vi "GUI_HTT_Cam_SubVI.vi"() -> (3 "image::2":T3(plugin-control))   [LabVIEW 2013]
uses:
  Shared/GUI_Template/GUI_master/tcp_new_data_event.ctl
  Shared/GUI_Template/GUI_master/tcp new data cluster.ctl
panel:
  in  "UDP error message":string
  out "tcp data event 2":T1
  out "error IO 2":errorcluster
  in  "active cams":string
  out "CCDs":string[](array[string])
  out "Cameras":T2
  in  "triggerdelay::2":dbl=0.001 caption="triggerdelay" min=0.0 max=10000.0 format="%_4p"
  in  "trigger::2":bool caption="Trigger"
  in  "exposure::2":dbl=0.001 caption="exposure" min=0.0001 max=1.0 format="%_4p"
  in  "GUIdevice 2":string="BellaCam13_4_gmode_s"
  out "tcp data event":T1
  in  "Refresh Button":bool caption="Update Crosshairs"
  in  "Select device":string(combo)="FrogHPD"
  in  "stop":bool
  in  "GUIdevice 1":string="HPD_CCD"
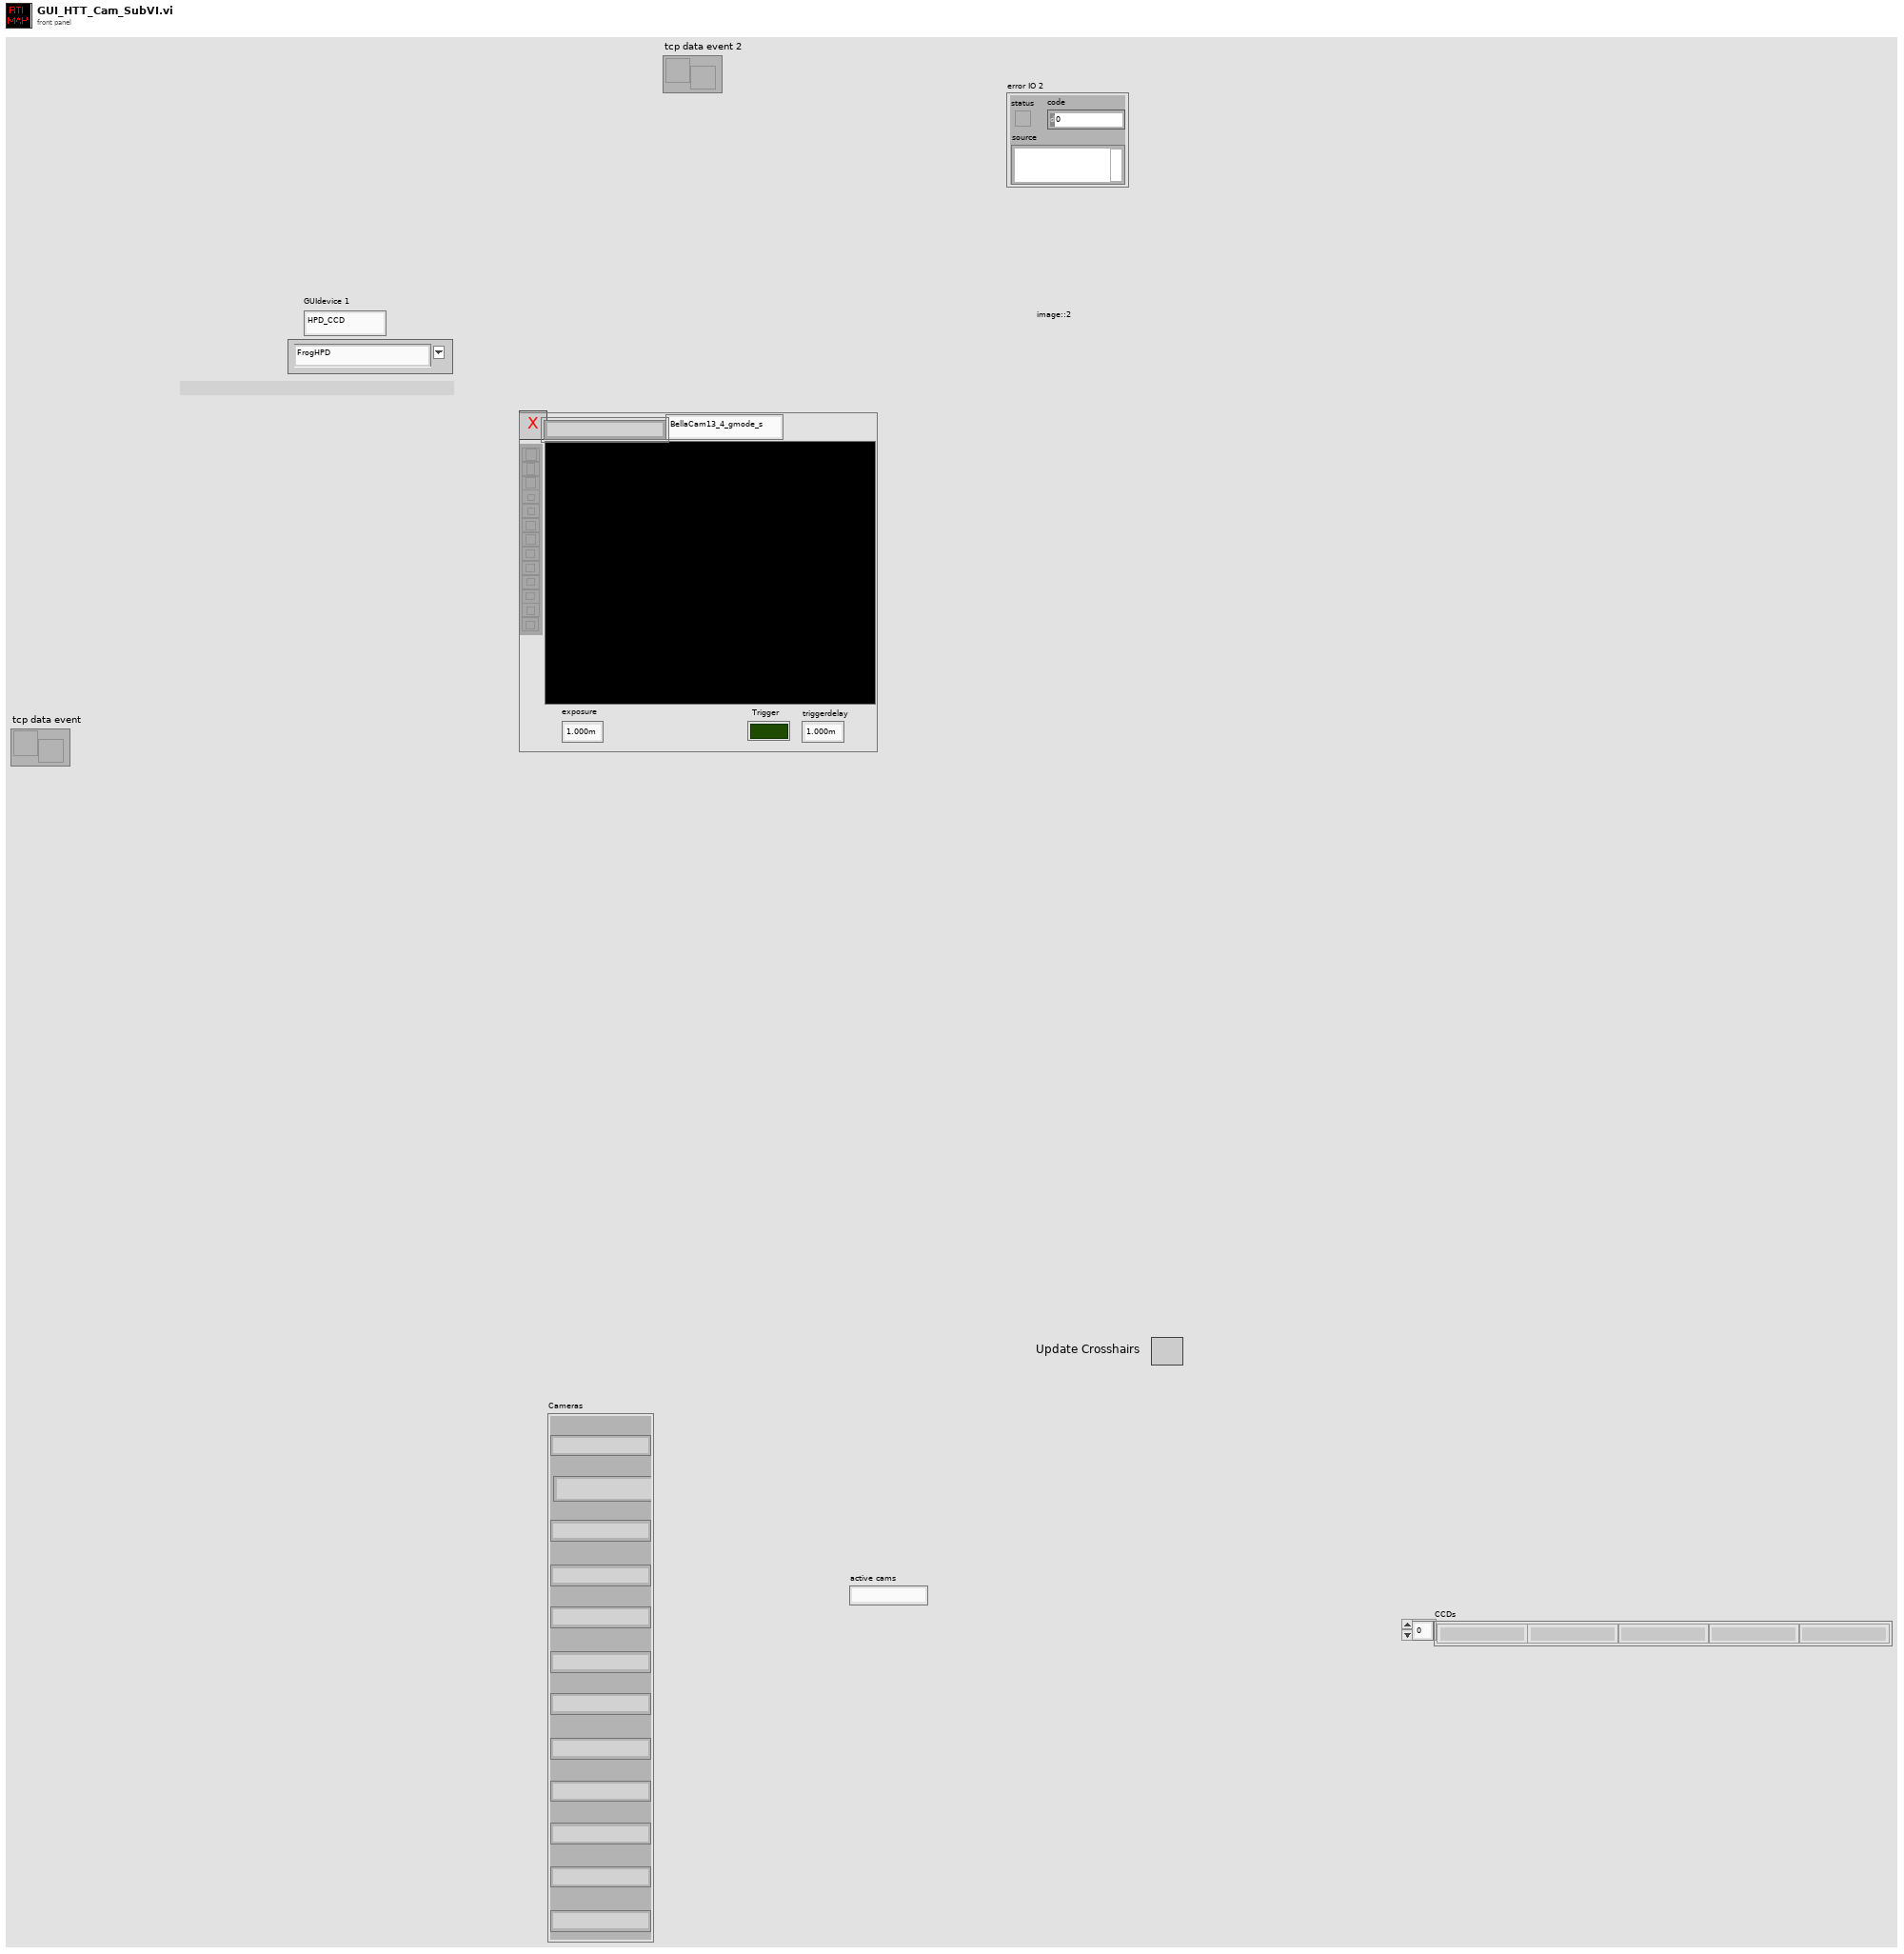
[diagram p1: front panel]
types:
  T1 = typedef "tcp_new_data_event.ctl" = refnum<user-event>
  T2 = cluster{"[0]":string, "[1]":string, "[2]":string, "[3]":string, "[4]":string, "[5]":string, "[6]":string, "[7]":string, "[8]":string, "[8] 2":string, "[8] 3":string, "[8] 4":string}
  T3 = typedef "IMAQ Image.ctl" = refnum<image>
  T4 = typedef "Image Type" = u32
  T5 = cluster{"[0]":string, "[1]":string, "[2]":string, "[3]":string, "[4]":string, "[5]":string, "[6]":string, "[7]":string, "[8]":string, "[9]":string, "[10]":string, "[11]":string}
  T6 = enum32{"invalid app kind", "Development System", "Run Time System", "Student Edition", "Embedded LabVIEW", "Evaluation", "Custom"}
  T7 = typedef "tcp new data cluster.ctl" = cluster{"EventEnum":enum16{"new data", "connection status update"}, "Device name":string}
  T8 = enum32{"Invalid", "Standard", "Closed", "Hidden", "Minimized", "Maximized"}
  T9 = cluster{"Core":cluster{"Current VI Reference":refnum<vi>, "Close Panel on Exit?":bool}, "Your Boolean data":bool, "active cams":string, "SuperGUI":cluster{"STOP queue":refnum<queue>, "SuperGUI ref":refnum<vi>}}
  T10 = cluster{"STOP queue":refnum<queue>, "SuperGUI ref":refnum<vi>}
  T11 = cluster{"Current VI Reference":refnum<vi>, "Close Panel on Exit?":bool}
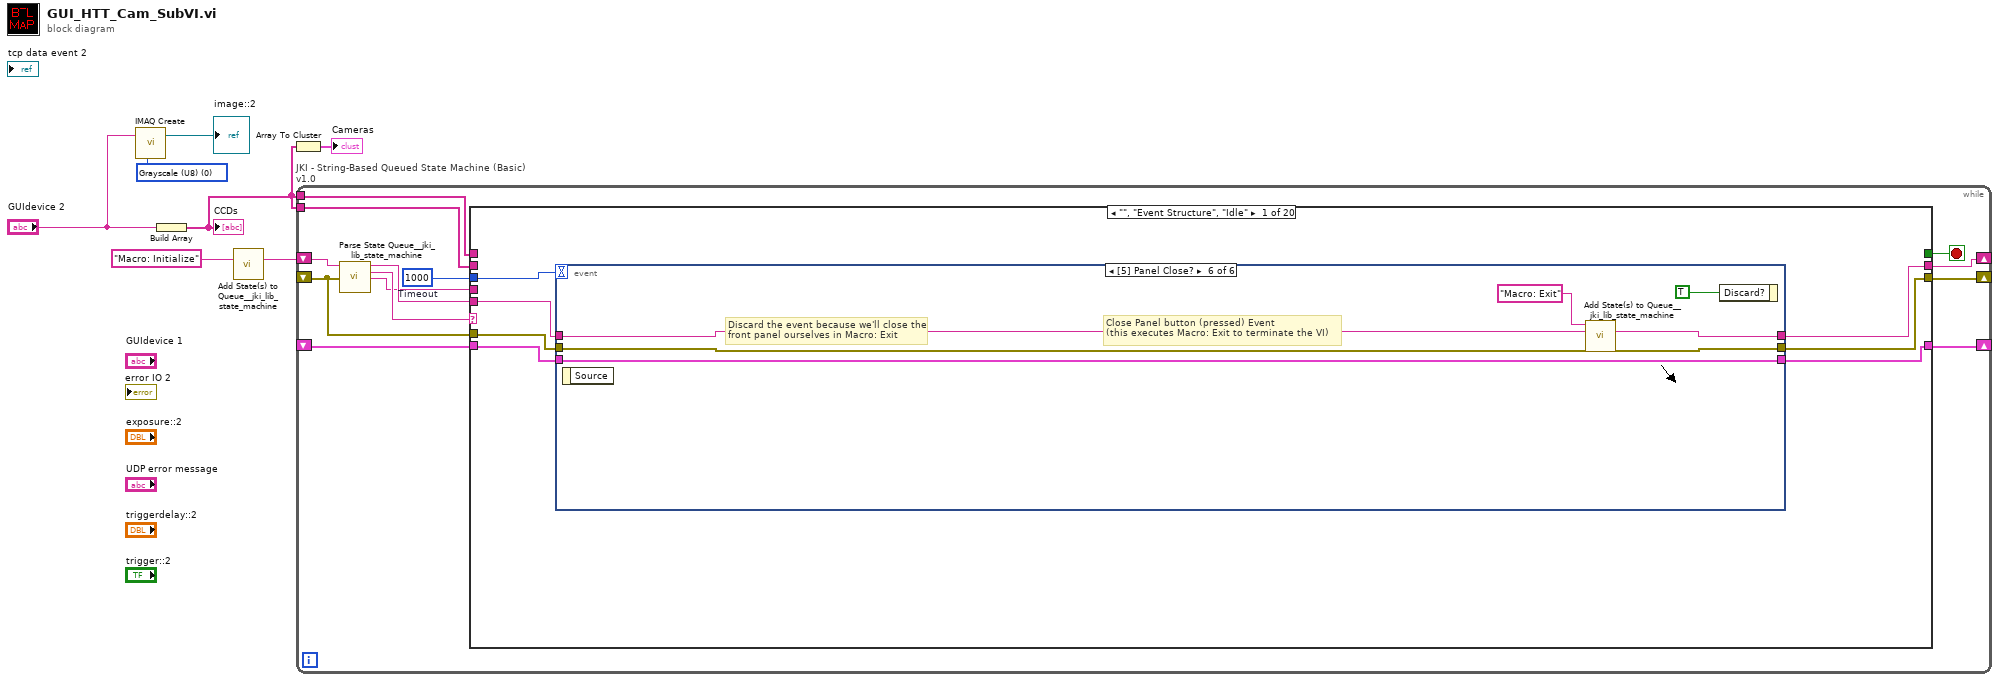
[diagram p0: block diagram]
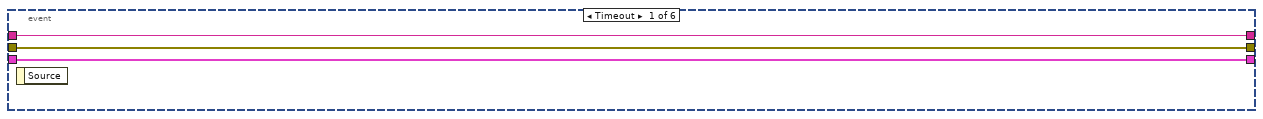
[diagram p2: hidden frame]
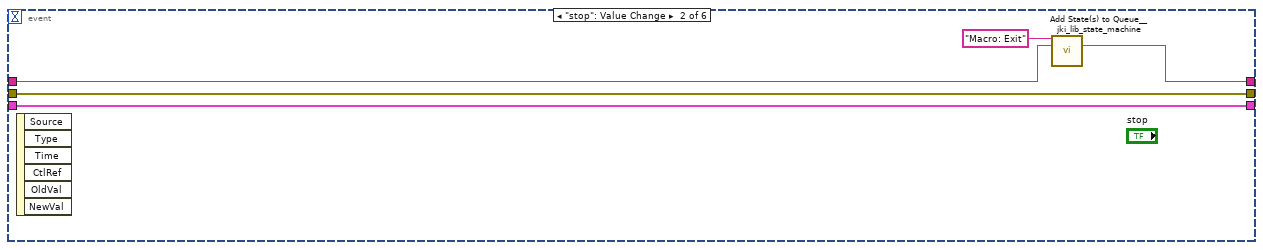
[diagram p3: hidden frame]
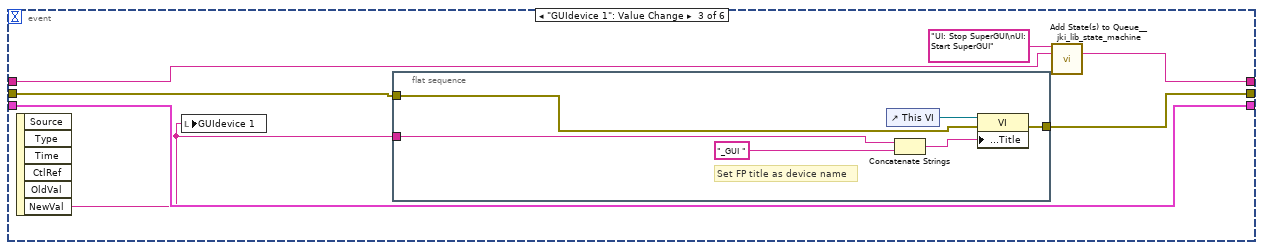
[diagram p4: hidden frame]
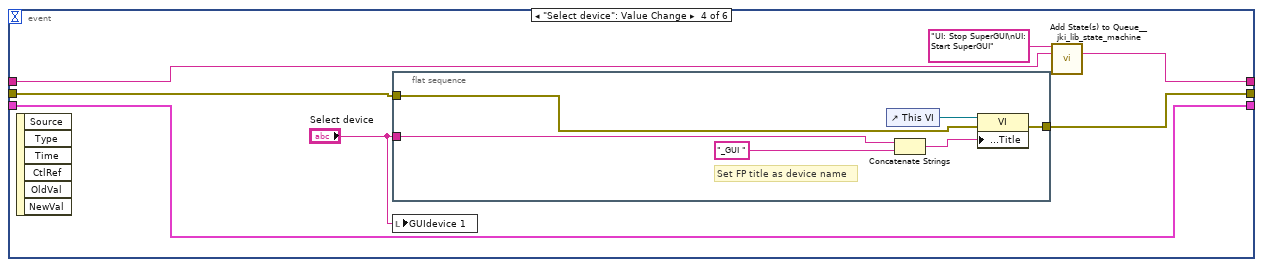
[diagram p5: hidden frame]
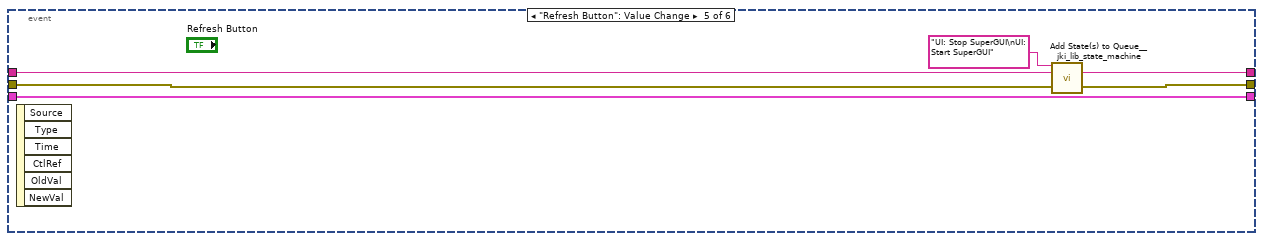
[diagram p6: hidden frame]
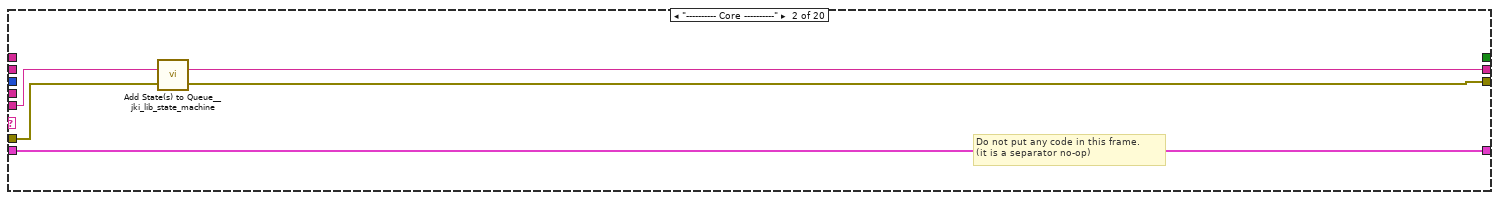
[diagram p7: hidden frame]
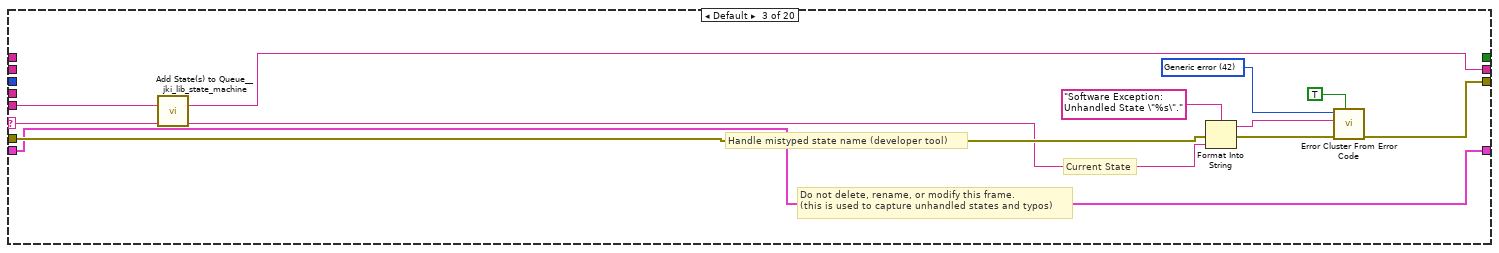
[diagram p8: hidden frame]
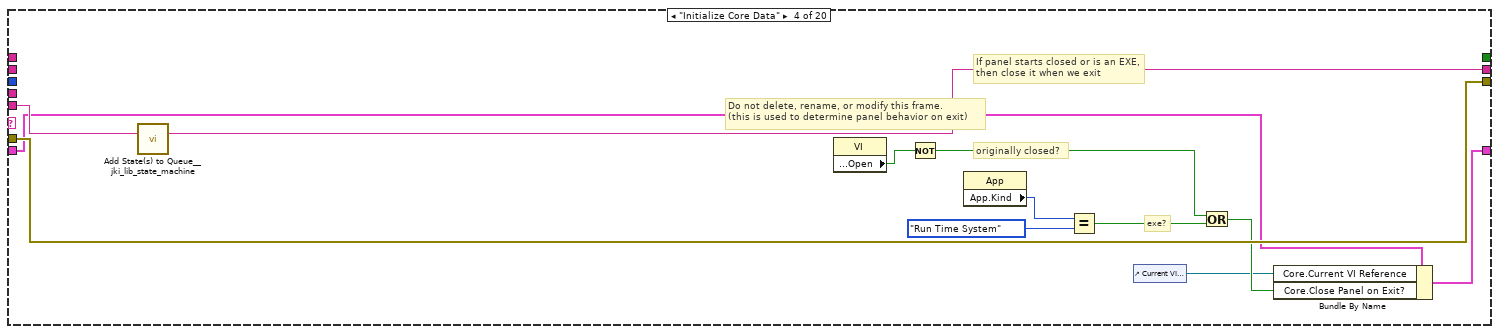
[diagram p9: hidden frame]
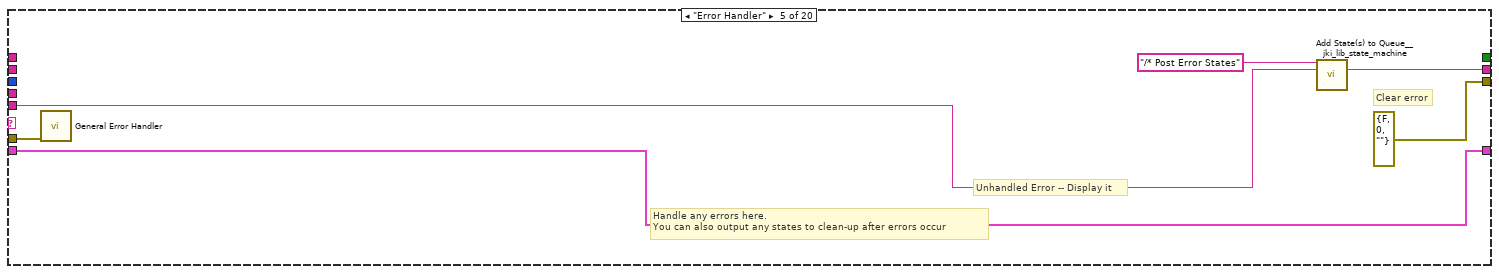
[diagram p10: hidden frame]
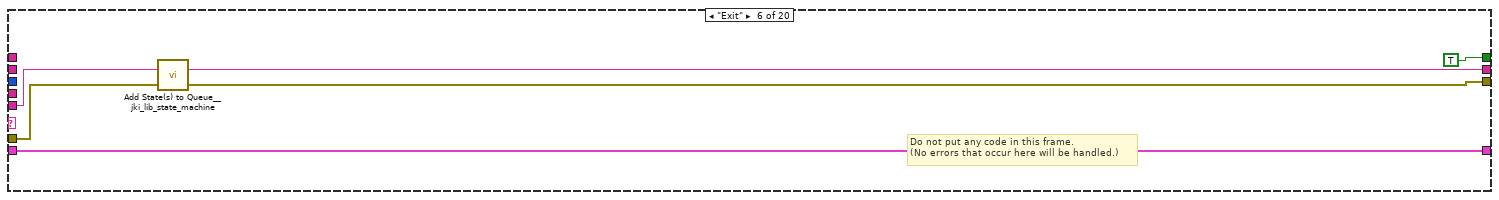
[diagram p11: hidden frame]
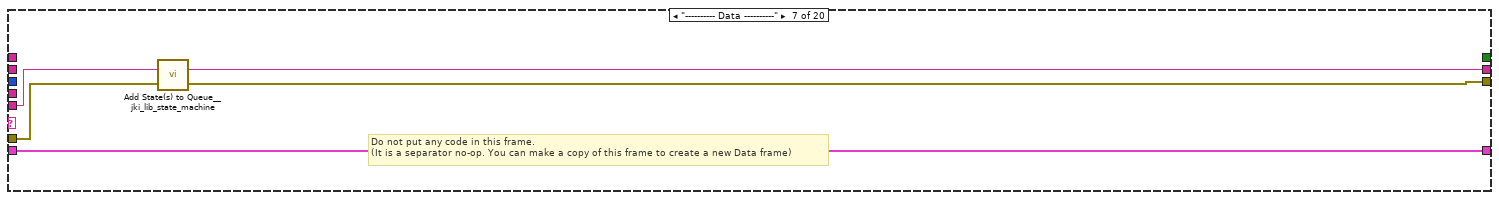
[diagram p12: hidden frame]
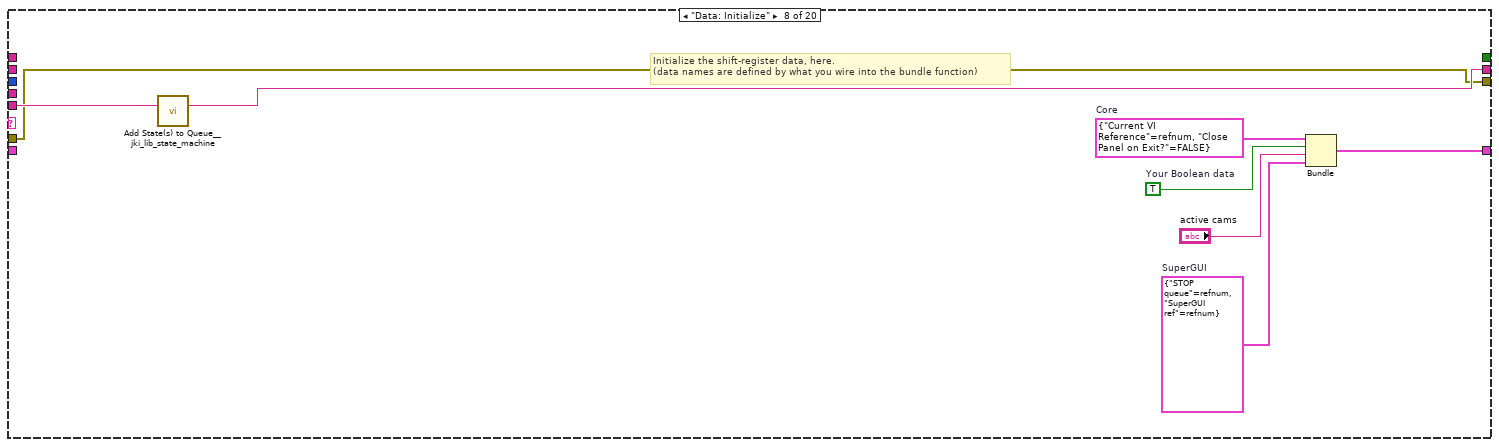
[diagram p13: hidden frame]
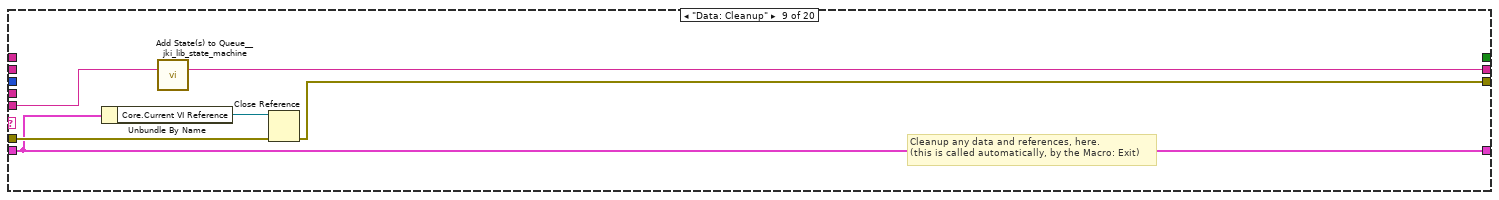
[diagram p14: hidden frame]
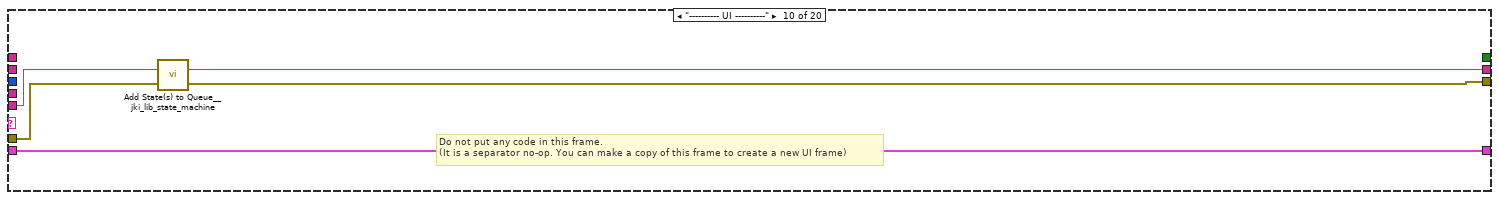
[diagram p15: hidden frame]
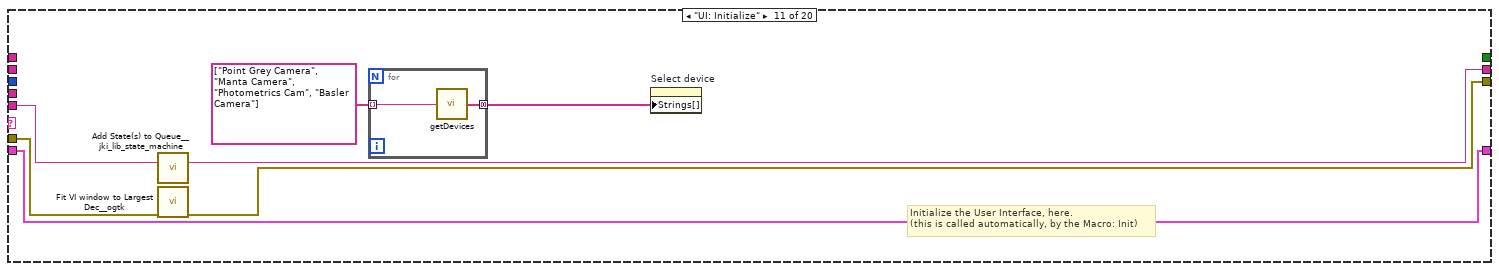
[diagram p16: hidden frame]
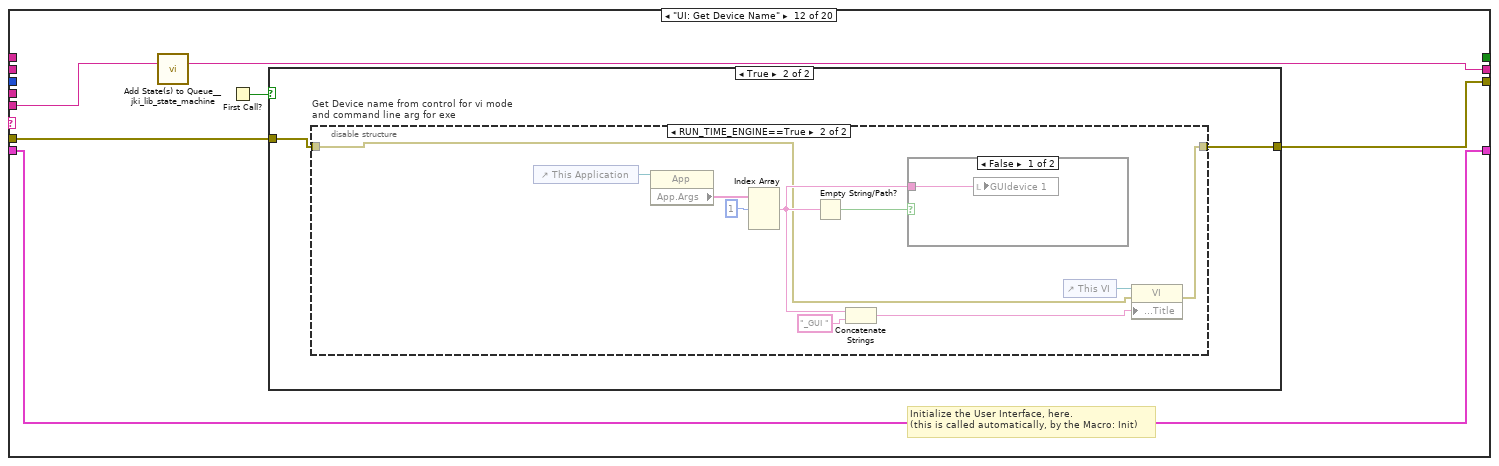
[diagram p17: hidden frame]
diagram:
  w1 = T4 0 items=["Grayscale (U8)", "Grayscale (I16)", "Grayscale (SGL)", "Complex (CSG)", "RGB (U32)", "HSL (U32)", "RGB (U64)", "Grayscale (U16)"] ("Image Type")
  n1 = call "IMAQ Create"("Image Name"="GUIdevice 2", "Image Type"=w1) -> ("New Image"=→"image::2":T3)  [unwired: 3 in, 1 out]
  n2 = Build Array("GUIdevice 2") -> (w2:string[])
  "CCDs" <- w2
  n3 = call <vilib>:"Add State(s) to Queue__jki_lib_state_machine.vi"("State(s) in (\"\")"="Macro: Initialize") -> ("States Out"=w7:string)  [unwired: 14 in]
  n4 = Array To Cluster(array=w2) -> (cluster=→"Cameras":T5)
  n5 = while "JKI - String-Based Queued State Machine (Basic) v1.0" {
    shift-right: [w13] -> _
    shift-left: _ -> [w10]
    shift-right: [w16] -> _
    shift-left: _ -> [w11]
    shift-right: [w15] -> _
    shift-left: w7 -> [w17]
    tunnel: w2 -> [w8]
    tunnel: w2 -> [w9]
    stop <- w14 stop-if-true
    w12 = 1000  # Timeout
    n6 = call <vilib>:"Parse State Queue__jki_lib_state_machine.vi"("State Queue"=w17, "Error In (no error)"=w11) -> ("Remaining States"=w19:string, "Current State"=w20:string, "Arguments"=w18:string)  [unwired: 11 in]
    n7 = case shown="\"\", \"Event Structure\", \"Idle\"" w20 {
      selector: w20 -> [_ _ w77 _ _ _ _ _ _ _ _ _ _ _ _ _ _ _ _ _]
      tunnel: w19 -> [w27 w76 w81 w99 w105 w110 w114 w122 w128 w132 w139 w147 w182 w190 w196 w207 w233 w238 w248 w252]
      tunnel: w18 -> [_ _ _ _ _ _ _ _ _ _ _ _ _ _ w191 w201 _ _ _ _]
      tunnel: w10 -> [w25 w73 w79 w90 w102 w108 w111 _ w123 w129 w137 w145 w173 w185 w194 w203 w230 w235 w245 w249]
      tunnel: [w24 w74 w83 w96 errorcluster {"status"=FALSE, "code"=0, "source"=""} ("error out") w107 w112 w119 w124 w130 w135 w142 w166 w183 w192 w204 w231 w236 w246 w250] -> w16
      tunnel: w11 -> [w23 w74 w82 w96 w101 w107 w112 w119 w125 w130 w136 w143 w167 w184 w193 w205 w231 w236 w246 w250]
      tunnel: [w26 w75 w80 w98 w104 w109 w113 w121 w127 w131 w138 w146 w181 w189 w195 w206 w232 w237 w247 w251] -> w15
      tunnel: [_ _ _ _ _ TRUE _ _ _ _ _ _ _ _ _ _ _ _ _ _] -> w14
      tunnel: [w22 w73 w79 w97 w102 w108 w111 w120 w123 w129 w137 w145 w172 w185 w194 w203 w230 w235 w245 w249] -> w13
      tunnel: w12 -> [w21 _ _ _ _ _ _ _ _ _ _ _ _ _ _ _ _ _ _ _]
      tunnel: w9 -> [_ _ _ _ _ _ _ _ _ _ _ _ _ _ _ _ _ _ _ _]
      tunnel: w8 -> [_ _ _ _ _ _ _ _ _ _ _ _ _ _ _ _ _ _ _ _]
      frame "", "Event Structure", "Idle" {
        n8 = event shown="[5] Panel Close?" {
          selector: _ -> [_ _ _ _ _ _]
          dyn-events: _ -> [_ _ _ _ _ _]
          timeout: w21 -> [_ _ _ _ _ _]
          tunnel: w27 -> [w28 w33 w39 w51 w64 w72]
          tunnel: [w28 w32 w38 w50 w63 w71] -> w26
          tunnel: w25 -> [w29 w35 w42 w55 w66 w69]
          tunnel: [w30 w34 w40 w53 w65 w70] -> w24
          tunnel: w23 -> [w30 w34 w41 w54 w65 w70]
          tunnel: [w29 w35 w42 w55 w66 w69] -> w22
          event Timeout {
            n9 = event-data() -> ()  [unwired: 1 in, 1 out]
          }
          event "stop": Value Change {
            n10 = event-data() -> ()  [unwired: 1 in, 6 out]
            n11 = call <vilib>:"Add State(s) to Queue__jki_lib_state_machine.vi"("State(s) in Front (\"\")"="Macro: Exit", "State(s) in (\"\")"=w33) -> ("States Out"=w32:string)  [unwired: 13 in]
          }
          event "GUIdevice 1": Value Change {
            n12 = event-data() -> ("NewVal"=w36:string)  [unwired: 1 in, 5 out]
            n13 = local write "GUIdevice 1"(w36) -> ()
            n14 = flat-sequence {
              tunnel: [w45] -> w40
              tunnel: w41 -> [w44]
              tunnel: w36 -> [w43]
              frame #0 {
                # "Set FP title as device name"
                n15 = control-ref of="This VI"() -> (w48:refnum<vi>)
                n16 = Concatenate Strings(w43, "_GUI ") -> (w47:string)
                n17 = property class="VI"(reference=w48, error in=w44, "Front Panel.Title"=w47) -> (error out=w45:errorcluster)  [unwired: 1 out]
              }
            }
            n18 = call <vilib>:"Add State(s) to Queue__jki_lib_state_machine.vi"("State(s) in Front (\"\")"="UI: Stop SuperGUI\nUI: Start SuperGUI", "State(s) in (\"\")"=w39) -> ("States Out"=w38:string)  [unwired: 13 in]
          }
          event "Select device": Value Change {
            n19 = event-data() -> ()  [unwired: 1 in, 6 out]
            n20 = flat-sequence {
              tunnel: [w58] -> w53
              tunnel: w54 -> [w57]
              tunnel: "Select device" -> [w56]
              frame #0 {
                # "Set FP title as device name"
                n21 = control-ref of="This VI"() -> (w61:refnum<vi>)
                n22 = Concatenate Strings(w56, "_GUI ") -> (w60:string)
                n23 = property class="VI"(reference=w61, error in=w57, "Front Panel.Title"=w60) -> (error out=w58:errorcluster)  [unwired: 1 out]
              }
            }
            n24 = local write "GUIdevice 1"("Select device") -> ()
            n25 = call <vilib>:"Add State(s) to Queue__jki_lib_state_machine.vi"("State(s) in Front (\"\")"="UI: Stop SuperGUI\nUI: Start SuperGUI", "State(s) in (\"\")"=w51) -> ("States Out"=w50:string)  [unwired: 13 in]
          }
          event "Refresh Button": Value Change {
            n26 = event-data() -> ()  [unwired: 1 in, 6 out]
            n27 = call <vilib>:"Add State(s) to Queue__jki_lib_state_machine.vi"("State(s) in Front (\"\")"="UI: Stop SuperGUI\nUI: Start SuperGUI", "State(s) in (\"\")"=w64) -> ("States Out"=w63:string)  [unwired: 13 in]
          }
          event Panel Close? {
            # "Discard the event because we'll close the front panel ourselves in Macro: Exit"
            # "Close Panel button (pressed) Event\n(this executes Macro: Exit to terminate the VI)"
            n28 = event-data() -> ()  [unwired: 1 in, 1 out]
            n29 = call <vilib>:"Add State(s) to Queue__jki_lib_state_machine.vi"("State(s) in Front (\"\")"="Macro: Exit", "State(s) in (\"\")"=w72) -> ("States Out"=w71:string)  [unwired: 13 in]
            n30 = event-data("Discard?"=TRUE) -> ()  [unwired: 1 in, 1 out]
          }
        }
      }
      frame "---------- Core ----------" {
        # "Do not put any code in this frame.\n(it is a separator no-op)"
        n31 = call <vilib>:"Add State(s) to Queue__jki_lib_state_machine.vi"("State(s) in (\"\")"=w76) -> ("States Out"=w75:string)  [unwired: 14 in]
      }
      frame Default {
        w86 = 42 items=["No error", "Argument error", "Memory is full", "Out of zone", "End of file", "File already open", "Generic file I/O error", "File not found", "File permission error", "Disk is full", "Duplicate path", "Too many files open", "System feature not enabled", "Resource file not found", "Cannot add resource", "Resource not found", "Image not found", "Image memory error", "Pen does not exist", "Config type invalid", "Config token not found", "Config parse error", "Config memory error", "Bad external code format", "Bad external code offset", "External code not present", "Null window", "Destroy window error", "Null menu", "Print aborted", "Bad print record", "Print driver error", "Windows error during printing", "Memory error during printing", "Print dialog error", "Generic print error", "Invalid device refnum", "Device not found", "Device parameter error", "Device unit error", "Cannot open device", "Device call aborted", "Generic error", "Cancelled by user", "Object ID too low", "Object ID too high", "Object not in heap", "Unknown heap", "Unknown object (invalid DefProc)", "Unknown object (DefProc not in table)", "Message out of range", "Invalid (null) method", "Unknown message", "Manager call not supported", "Bad address", "Network operation in progress", "Network operation timed out", "Connection is busy", "Network attribute not supported", "Network error", "Address in use", "System out of memory", "Connection aborted", "Connection refused", "Not connected", "Already connected", "Connection closed", "Initialization error (interapplication manager)", "Bad occurrence", "Wait on unbound occurrence handler", "Occurrence queue overflow", "Datalog type conflict", "Unused", "Unrecognized type (interapplication manager)", "Memory corrupt", "Failed to make temporary DLL", "Old CIN version", "Drag socket not found", "Failed to load drop-object", "Failed to register OLE object", "Failed to release OLE object", "Format specifier type mismatch", "Unknown format specifier", "Too few format specifiers", "Too many format specifiers", "Scan failed", "Newer CIN version", "Error converting to variant", "Runtime menu error", "Password tampered", "Variant attribute not found", "Incompatible variant data type", "Event data is not available", "Event Store is not present", "Occurrence is not found", "Event Queue is not created", "Event info is not available", "Refnum passed is NULL", "Error retrieving Class GUID", "Error retrieving CoClass GUID", "Error retrieving TypeLib GUID.", "Bad built application magic bytes.", "Specific driver is different from the specific driver associated with the Logical Name.", "There is no session opened to the class driver.", "Max Error", "MAX - Error with config objects", "MAX - Error loading configuration", "MAX - Group not supported"]
        # "Current State"
        # "Do not delete, rename, or modify this frame.\n(this is used to capture unhandled states and typos)"
        # "Handle mistyped state name (developer tool)"
        n32 = call <vilib>:"Add State(s) to Queue__jki_lib_state_machine.vi"("State(s) in (\"\")"=w81) -> ("States Out"=w80:string)  [unwired: 14 in]
        n33 = Format Into String(format string="Software Exception: Unhandled State \"%s\"." ("message"), error in=w82, w77) -> (resulting string=w85:string, error out=w84:errorcluster)  [unwired: 1 in]
        n34 = call <vilib>:"Error Cluster From Error Code.vi"("show call chain? (False)"=TRUE, "error in (no error)"=w84, "error message (\"\")"=w85, "error code (0)"=w86) -> ("error out"=w83:errorcluster)  [unwired: 5 in]
      }
      frame "Initialize Core Data" {
        # "Do not delete, rename, or modify this frame.\n(this is used to determine panel behavior on exit)"
        # "originally closed?"
        # "exe?"
        # "If panel starts closed or is an EXE, then close it when we exit"
        n35 = call <vilib>:"Add State(s) to Queue__jki_lib_state_machine.vi"("State(s) in (\"\")"=w99) -> ("States Out"=w98:string)  [unwired: 14 in]
        n36 = property class="VI"() -> ("Front Panel.Open"=w95:bool)  [unwired: 2 in, 2 out]
        n37 = Not(x=w95) -> (.not. x?=w92:bool)
        n38 = property class="App"() -> ("App.Kind"=w94:T6)  [unwired: 2 in, 2 out]
        n39 = Equal?(x=w94, y=T6."Run Time System" ("Application:Kind")) -> (x = y?=w91:bool)
        n40 = control-ref of="Current VI Reference"() -> (w88:refnum<vi>)
        n41 = Or(x=w92, y=w91) -> (x .or. y?=w89:bool)
        n42 = Bundle By Name(cluster=w90, "Core.Current VI Reference"=w88, "Core.Close Panel on Exit?"=w89) -> (w97:T9)
      }
      frame "Error Handler" {
        # "Unhandled Error -- Display it"
        # "Handle any errors here.\nYou can also output any states to clean-up after errors occur"
        # "Clear error"
        n43 = call <vilib>:"General Error Handler.vi"("error in (no error)"=w101) -> ()  [unwired: 10 in, 5 out]
        n44 = call <vilib>:"Add State(s) to Queue__jki_lib_state_machine.vi"("State(s) in Front (\"\")"="/* Post Error States", "State(s) in (\"\")"=w105) -> ("States Out"=w104:string)  [unwired: 13 in]
      }
      frame "Exit" {
        # "Do not put any code in this frame.\n(No errors that occur here will be handled.)"
        n45 = call <vilib>:"Add State(s) to Queue__jki_lib_state_machine.vi"("State(s) in (\"\")"=w110) -> ("States Out"=w109:string)  [unwired: 14 in]
      }
      frame "---------- Data ----------" {
        # "Do not put any code in this frame.\n(It is a separator no-op. You can make a copy of this frame to create a new Data frame)"
        n46 = call <vilib>:"Add State(s) to Queue__jki_lib_state_machine.vi"("State(s) in (\"\")"=w114) -> ("States Out"=w113:string)  [unwired: 14 in]
      }
      frame "Data: Initialize" {
        w115 = T10 {"STOP queue"=refnum, "SuperGUI ref"=refnum}  # SuperGUI
        w116 = T11 {"Current VI Reference"=refnum, "Close Panel on Exit?"=FALSE}  # Core
        w118 = TRUE  # Your Boolean data
        # "Initialize the shift-register data, here.\n(data names are defined by what you wire into the bundle function)"
        n47 = call <vilib>:"Add State(s) to Queue__jki_lib_state_machine.vi"("State(s) in (\"\")"=w122) -> ("States Out"=w121:string)  [unwired: 14 in]
        n48 = Bundle("Core"=w116, "Your Boolean data"=w118, "active cams"="active cams", "SuperGUI"=w115) -> (w120:T9)  [unwired: 1 in]
      }
      frame "Data: Cleanup" {
        # "Cleanup any data and references, here.\n(this is called automatically, by the Macro: Exit)"
        n49 = Unbundle By Name(w123) -> ("Core.Current VI Reference"=w126:refnum<vi>)
        n50 = call <vilib>:"Add State(s) to Queue__jki_lib_state_machine.vi"("State(s) in (\"\")"=w128) -> ("States Out"=w127:string)  [unwired: 14 in]
        n51 = Close Reference(reference=w126, error in (no error)=w125) -> (error out=w124:errorcluster)
      }
      frame "---------- UI ----------" {
        # "Do not put any code in this frame.\n(It is a separator no-op. You can make a copy of this frame to create a new UI frame)"
        n52 = call <vilib>:"Add State(s) to Queue__jki_lib_state_machine.vi"("State(s) in (\"\")"=w132) -> ("States Out"=w131:string)  [unwired: 14 in]
      }
      frame "UI: Initialize" {
        # "Initialize the User Interface, here.\n(this is called automatically, by the Macro: Init)"
        n53 = call <vilib>:"Add State(s) to Queue__jki_lib_state_machine.vi"("State(s) in (\"\")"=w139) -> ("States Out"=w138:string)  [unwired: 14 in]
        n54 = call <userlib>:"Fit VI window to Largest Dec__ogtk.vi"("error in (no error)"=w136) -> ("error out"=w135:errorcluster)  [unwired: 5 in, 1 out]
        n55 = for {
          tunnel: string[] ["Point Grey Camera", "Manta Camera", "Photometrics Cam", "Basler Camera"] -> [w141] mode=indexing
          tunnel: [w140] -> w133 mode=concatenating
          n56 = call "getDevices.vi"("Device Class"=w141) -> ("All Devices"=w140:string[])
        }
        n57 = property on="Select device" class="CmbBox"("Strings[]"=w133) -> ()  [unwired: 2 in, 2 out]
      }
      frame "UI: Get Device Name" {
        # "Initialize the User Interface, here.\n(this is called automatically, by the Macro: Init)"
        n58 = call <vilib>:"Add State(s) to Queue__jki_lib_state_machine.vi"("State(s) in (\"\")"=w147) -> ("States Out"=w146:string)  [unwired: 14 in]
        n59 = First Call?() -> (First Call?: T/F=w144:bool)
        n60 = case shown="True" w144 {
          tunnel: w143 -> [w148 w150]
          tunnel: [w148 w149] -> w142
          frame False {
          }
          frame True {
            n61 = disable-structure "Get Device name from control for vi mode\nand command line arg for exe" shown="RUN_TIME_ENGINE==True" {
              disable-tunnel: w150 -> [w151 w153]
              disable-tunnel: [w151 w152] -> w149
              frame condition #0 (active) {
              }
              frame condition #1 {
                n62 = control-ref of="This Application"() -> (w161:refnum<vi>)
                n63 = property class="App"(reference=w161) -> ("App.Args"=w160:string[])  [unwired: 1 in, 2 out]
                n64 = Index Array(array=w160, index #1=1 ("index")) -> (element #1=w154:string)  [unwired: 2 in, 2 out]
                n65 = Empty String/Path?(string/path=w154) -> (empty?=w158:bool)
                n66 = Concatenate Strings(w154, "_GUI ") -> (w156:string)
                n67 = case shown="False" w158 {
                  tunnel: w154 -> [w162 _]
                  frame False {
                    n68 = local write "GUIdevice 1"(w162) -> ()
                  }
                  frame True {
                  }
                }
                n69 = control-ref of="This VI"() -> (w157:refnum<vi>)
                n70 = property class="VI"(reference=w157, error in=w153, "Front Panel.Title"=w156) -> (error out=w152:errorcluster)  [unwired: 1 out]
              }
            }
          }
        }
      }
      frame "UI: Start SuperGUI" {
        # "create stop queue for supergui and its clones"
        # "x100 abort will be dependent on caller VI\nx80 abort will be independent of caller vi, this will abort vi when labview is closed."
        # "Start SuperGUI asynchronous way"
        n71 = vi-ref "GUI_Master_subvi_reentrant_queues.vi"() -> (w165:refnum<vi>)
        n72 = property class="VI"(reference=w165) -> ("Path"=w164:path)  [unwired: 1 in, 2 out]
        n73 = control-ref of="This Application"() -> (w171:refnum<vi>)
        n74 = Open VI Reference(type specifier VI Refnum (for type only)=refnum<vi> refnum, vi path=w164, options=256) -> (vi reference=w180:refnum<vi>, error out=w179:errorcluster)  [unwired: 3 in]
        n75 = Create User Event(user event datatype=T7 {"EventEnum"=enum."new data", "Device name"="Device name"} ("New Event"), error in=w167) -> (user event=w168:refnum<user-event>, error out=w174:errorcluster)
        "tcp data event" <- w168
        n76 = register-events(w168) -> ()  [unwired: 2 in, 2 out]
        n77 = control-ref of="This VI"() -> (w170:refnum<vi>)
        n78 = call "supergui create stop queue.vi"() -> ("STOP Queue out"=w176:refnum<queue>)  [unwired: 11 in]
        n79 = Current VI's Menubar() -> (w169:refnum<k9>)
        n80 = call-by-ref "Start Asynchronous Call"(reference=w180, error in=w179, "STOP Queue in"=w176, "This Application"=w171, 8:"error in (no error)"=w174, "tcp data event"=w168, "Caller menu reference"=w169, "Caller VI ref"=w170) -> (reference out=w163:refnum<vi>, error out=w166:errorcluster)  [unwired: 5 in, 1 out]
        n81 = Bundle By Name(cluster=w173, "SuperGUI.SuperGUI ref"=w163, "SuperGUI.STOP queue"=w176) -> (w172:T9)
        n82 = call <vilib>:"Add State(s) to Queue__jki_lib_state_machine.vi"("State(s) in (\"\")"=w182) -> ("States Out"=w181:string)  [unwired: 14 in]
      }
      frame "UI: Stop SuperGUI" {
        # "Stop Supergui Clone and wait until it exit properly"
        n83 = call <vilib>:"Add State(s) to Queue__jki_lib_state_machine.vi"("State(s) in (\"\")"=w190) -> ("States Out"=w189:string)  [unwired: 14 in]
        n84 = Unbundle By Name(w185) -> ("SuperGUI.SuperGUI ref"=w187:refnum<vi>, "SuperGUI.STOP queue"=w186:refnum<queue>)
        n85 = Release Queue(queue=w186, error in (no error)=w184) -> (error out=w188:errorcluster)  [unwired: 1 in, 2 out]
        n86 = call-by-ref "Wait On Asynchronous Call"(reference=w187, error in=w188) -> ("error out"=w183:errorcluster)  [unwired: 11 in, 2 out]
      }
      frame "UI: Cursor Set" {
        # "Argument"
        # "Set and Unset Cursor Busy.\n(Usage: \"UI: Cursor Set >> Busy|Idle\")"
        n87 = call <vilib>:"Add State(s) to Queue__jki_lib_state_machine.vi"("State(s) in (\"\")"=w196) -> ("States Out"=w195:string)  [unwired: 14 in]
        n88 = case shown="\"Idle\", Default" w191 {
          tunnel: w193 -> [w198 w200]
          tunnel: [w197 w199] -> w192
          frame "Idle", Default {
            n89 = call <vilib>:"Unset Busy.vi"("error in (no error)"=w198) -> ("error out"=w197:errorcluster)  [unwired: 10 in]
          }
          frame "Busy" {
            n90 = call <vilib>:"Set Busy.vi"("error in (no error)"=w200) -> ("error out"=w199:errorcluster)  [unwired: 9 in, 1 out]
          }
        }
      }
      frame "UI: Front Panel State" {
        # "Argument"
        # "Set Front Panel Open or Closed\n(Usage: \"UI: Front Panel State >> Open|Close\")"
        n91 = call <vilib>:"Add State(s) to Queue__jki_lib_state_machine.vi"("State(s) in (\"\")"=w207) -> ("States Out"=w206:string)  [unwired: 14 in]
        n92 = Unbundle By Name(w203) -> ("Core.Current VI Reference"=w202:refnum<vi>)
        n93 = case shown="\"Open\", Default" w201 {
          tunnel: w205 -> [w211 w224]
          tunnel: [w213 w225] -> w204
          tunnel: w202 -> [w212 w222]
          frame "Open", Default {
            n94 = property class="VI"(reference=w212, error in=w211) -> (reference out=w209:refnum<vi>, error out=w210:errorcluster, "Front Panel.Open"=w208:bool)
            n95 = case shown="False" w208 {
              tunnel: [w216 w219] -> w213
              tunnel: w210 -> [w215 w219]
              tunnel: w209 -> [w214 _]
              frame False {
                n96 = invoke class="VI" method="FP.Open"(reference=w214, error in=w215, "Activate"=TRUE, "State"=T8."Standard") -> (error out=w216:errorcluster)  [unwired: 1 in, 4 out]
              }
              frame True {
              }
            }
          }
          frame "Close" {
            n97 = property class="VI"(reference=w222, error in=w224) -> (reference out=w221:refnum<vi>, error out=w223:errorcluster, "Front Panel.Open"=w220:bool)
            n98 = case shown="True" w220 {
              tunnel: [w226 w229] -> w225
              tunnel: w223 -> [w226 w228]
              tunnel: w221 -> [_ w227]
              frame False {
              }
              frame True {
                n99 = invoke class="VI" method="FP.Close"(reference=w227, error in=w228) -> (error out=w229:errorcluster)  [unwired: 1 in, 2 out]
              }
            }
          }
        }
      }
      frame "---------- Macro ----------" {
        # "Do not put any code in this frame.\n(It is a separator no-op. You can make a copy of this frame to create a new Macro frame)"
        n100 = call <vilib>:"Add State(s) to Queue__jki_lib_state_machine.vi"("State(s) in (\"\")"=w233) -> ("States Out"=w232:string)  [unwired: 14 in]
      }
      frame "Macro: Initialize" {
        # "Initialization Macro\n(This is called once, when the VI starts)"
        n101 = call <vilib>:"Add State(s) to Queue__jki_lib_state_machine.vi"("State(s) in Front (\"\")"="Data: Initialize\nInitialize Core Data\nUI: Initialize\nUI: Get Device Name\nUI: Start SuperGUI\nUI: Front Panel State >> Open", "State(s) in (\"\")"=w238) -> ("States Out"=w237:string)  [unwired: 13 in]
      }
      frame "Macro: Exit" {
        # "Exit Macro\n(This is called once, when the VI exits)"
        n102 = Unbundle By Name(w245) -> ("Core.Close Panel on Exit?"=w244:bool)
        n103 = Select(t="UI: Front Panel State >> Close", s=w244, f="") -> (s? t:f=w241:string)
        n104 = call <vilib>:"Add State(s) to Queue__jki_lib_state_machine.vi"("State(s) in (\"\")"=w241, "State(s) at Back (\"\")"="Data: Cleanup\nExit") -> ("States Out"=w239:string)  [unwired: 13 in]
        n105 = call <vilib>:"Add State(s) to Queue__jki_lib_state_machine.vi"("State(s) in Front (\"\")"=w239, "State(s) in (\"\")"=w248) -> ("States Out"=w247:string)  [unwired: 13 in]
      }
      frame "---------- New Category ----------" {
        # "Template Separator\n(You can make a copy of, or modify, this frame)"
        n106 = call <vilib>:"Add State(s) to Queue__jki_lib_state_machine.vi"("State(s) in (\"\")"=w252) -> ("States Out"=w251:string)  [unwired: 14 in]
      }
    }
  }
